vi "Kinect Statusvi.vi"(8 "error in (no error)":errorcluster, 11 "Kinect":i32) -> (0 "error out":errorcluster, 2 "Conectado":bool, 3 "Status":i32(ring) items=["Undefined", "Disconnected", "Connected", "Initializing", "Error", "NotPowered", "NotReady", "DeviceNotGenuine", "DeviceNotSupported", "InsufficientBandwidth"])   [LabVIEW 2016]
uses:
  Microsoft.Kinect
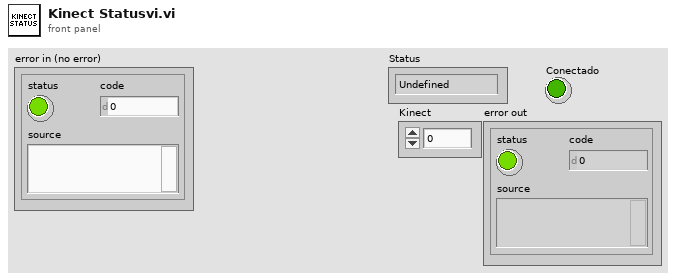
[diagram p1: front panel]
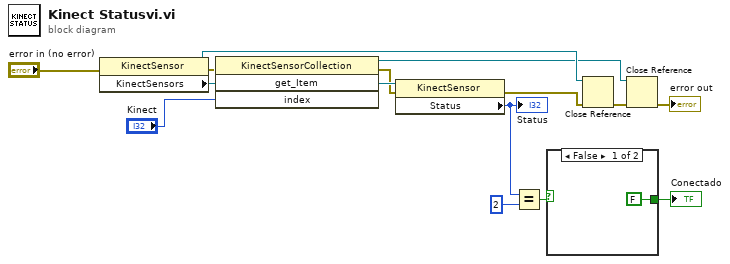
[diagram p0: block diagram]
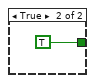
[diagram p2: hidden frame]
diagram:
  n1 = property class="KinectSensor"(error in="error in (no error)") -> (reference out=w12:refnum<k24>, error out=w7:errorcluster, "KinectSensors"=w15:refnum<k24>)  [unwired: 1 in]
  n2 = invoke class="KinectSensorCollection" method="get_Item"(reference=w15, error in=w7, "index"="Kinect") -> (reference out=w10:refnum<k24>, error out=w8:errorcluster, "get_Item"=w13:refnum<k24>)  [unwired: 1 in, 1 out]
  n3 = property class="KinectSensor"(reference=w13, error in=w8) -> (error out=w9:errorcluster, "Status"=w5:i32)  [unwired: 1 out]
  "Status" <- w5
  n4 = Equal?(x=w5, y=2) -> (x = y?=w3:bool)
  n5 = case shown="False" w3 {
    tunnel: [FALSE TRUE] -> w2
    frame False {
    }
    frame True {
    }
  }
  "Conectado" <- w2
  n6 = Close Reference(reference=w12, error in (no error)=w9) -> (error out=w11:errorcluster)
  n7 = Close Reference(reference=w10, error in (no error)=w11) -> (error out=→"error out":errorcluster)
